vi "get status.vi"(8 "error in (no error)":errorcluster, 11 "Camera":T1) -> (0 "error out":errorcluster, 2 "Error List":map{string, u64}(c390), 3 "Camera out":T1)   [LabVIEW 2024, in "Vision.lvlib"]
uses:
  Vision.lvlib
  camera.ctl
  camera driver.ctl
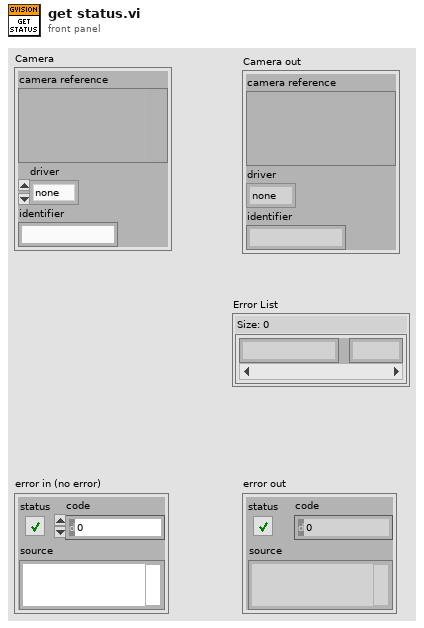
[diagram p1: front panel]
types:
  T1 = typedef "Vision.lvlib/camera.ctl" = cluster{"camera reference":variant, "driver":T2, "identifier":string}
  T2 = typedef "Vision.lvlib/camera driver.ctl" = enum16{"none", "wmf", "imaqdx", "peak"}
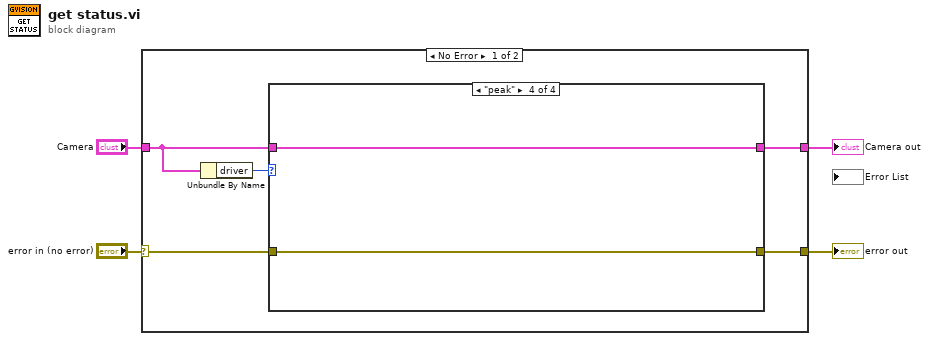
[diagram p0: block diagram]
diagram:
  n1 = case shown="No Error" "error in (no error)" {
    selector: "error in (no error)" -> [w7 w19]
    tunnel: [w8 w19] -> w3
    tunnel: "Camera" -> [w6 w18]
    tunnel: [w5 w18] -> w1
    frame No Error {
      n2 = Unbundle By Name(w6) -> ("driver"=w9:T2)
      n3 = case shown="\"peak\"" w9 {
        tunnel: w7 -> [w11 w13 w14 w16]
        tunnel: [w11 w13 w14 w16] -> w8
        tunnel: w6 -> [w10 w12 w15 w17]
        tunnel: [w10 w12 w15 w17] -> w5
        frame "none" {
        }
        frame "wmf" {
        }
        frame "imaqdx" {
        }
        frame "peak" {
        }
      }
    }
    frame Error {
    }
  }
  "error out" <- w3
  "Camera out" <- w1
